vi "Init.vi"(8 "error in (no error)":errorcluster) -> (0 "error out":errorcluster, 3 "Service Container out":refnum<class "Service Container.lvclass">)   [LabVIEW 2020, in "Vecto.lvlib" / "Service Container.lvclass"]
uses:
  Service Container.lvclass
  Services.ctl
  Service/Service.lvclass
  Service Container.lvclass/Service Container.ctl
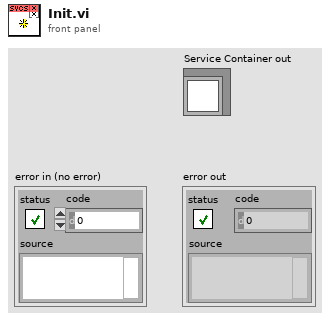
[diagram p1: front panel]
types:
  T1 = typedef "Vecto.lvlib/Service Container.lvclass/Services.ctl" = map{string, map{string, refnum<class "Service.lvclass">}}
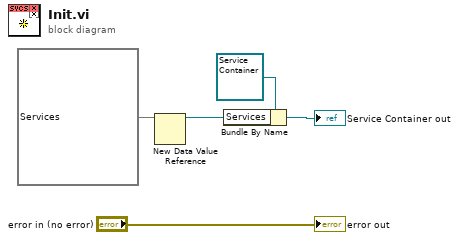
[diagram p0: block diagram]
diagram:
  n1 = New Data Value Reference(data value=T1 {} ("Services")) -> (data value reference=w1:refnum<data-value>)  [unwired: 1 in, 1 out]
  n2 = Bundle By Name(cluster=refnum<class "Service Container.lvclass"> refnum ("Service Container in"), "Services"=w1) -> (→"Service Container out":refnum<class "Service Container.lvclass">)
  "error out" <- "error in (no error)"
